vi "poly_fit.vi"(0 "y":dbl[](array[numeric]), 1 "order":i32, 5 "x":dbl[](array[numeric])) -> (4 "P(A)":dbl[](array[numeric]), 6 "P(x)":dbl[](array[numeric]), 15 "error":i32)   [LabVIEW 2020]
uses:
  <vilib>/Analysis/Matrix/Numeric/Conversions/Array To Matrix - RA.vi
  <vilib>/Analysis/Matrix/Numeric/Conversions/Array To Matrix - RA2.vi
  <vilib>/Analysis/Matrix/Numeric/Multiply/Multiply - RM,RM.vi
  <vilib>/Analysis/baseanly.llb/Real Inverse Matrix.vi
  <vilib>/Analysis/Matrix/Numeric/Conversions/Matrix To Array - RM.vi
  <vilib>/Analysis/Matrix/NI_Matrix.lvlib
  <vilib>/Analysis/NI_AALBase.lvlib
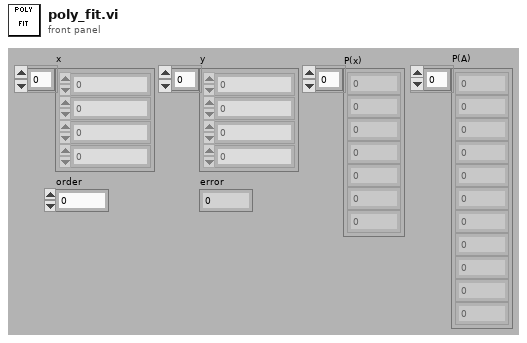
[diagram p1: front panel]
types:
  T1 = typedef "NI_Matrix.lvlib/RealMatrix.ctl" = dbl[][]
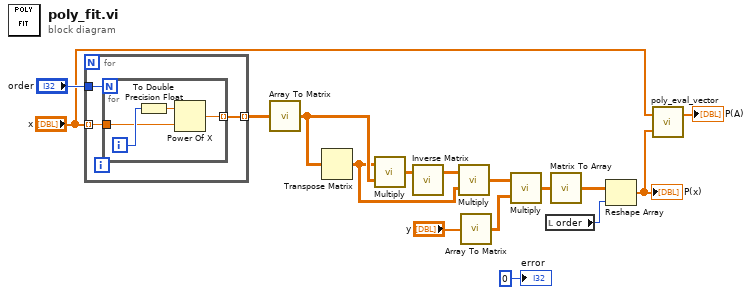
[diagram p0: block diagram]
diagram:
  n1 = for {
    tunnel: "x" -> [w19] mode=indexing
    tunnel: [w18] -> w16 mode=indexing
    tunnel: "order" -> [w17]
    n2 = for {
      N: w17 -> [_]
      tunnel: w19 -> [w21]
      tunnel: [w20] -> w18 mode=indexing
      i -> [w22]
      n3 = To Double Precision Float(number=w22) -> (double precision float=w23:dbl)
      n4 = Power Of X(1:w21, 2:w23) -> (0:w20:dbl)
    }
  }
  n5 = call-poly <vilib>:"Array To Matrix.vi"("Real 2D Array"=w16) -> ("Real Matrix"=w15:T1)
  n6 = Transpose Matrix(1:w15) -> (0:w12:T1)
  n7 = call-poly <vilib>:"Multiply.vi"("Real Matrix B"=w15, "Real Matrix A"=w12) -> ("A * B"=w14:T1)
  n8 = call-poly <vilib>:"Inverse Matrix.vi"("Input Matrix"=w14) -> ("Inverse Matrix"=w13:T1)  [unwired: 1 in, 1 out]
  n9 = call-poly <vilib>:"Multiply.vi"("Real Matrix B"=w12, "Real Matrix A"=w13) -> ("A * B"=w10:T1)
  n10 = call-poly <vilib>:"Array To Matrix.vi"("Real 1D Array"="y") -> ("Real Matrix (Column Vector)"=w9:T1)
  n11 = call-poly <vilib>:"Multiply.vi"("Real Matrix B"=w9, "Real Matrix A"=w10) -> ("A * B"=w8:T1)
  n12 = local read "order"() -> (w5:i32)
  n13 = call-poly <vilib>:"Matrix To Array.vi"("Real Matrix"=w8) -> ("Real 2D Array"=w6:dbl[][])
  n14 = Reshape Array(w6, w5) -> (w4:dbl[])
  "P(x)" <- w4
  n15 = call "poly_eval_vector.vi"("P(x)"=w4, "A"="x") -> ("P(A)"=→"P(A)":dbl[])  [unwired: 1 in]
  "error" <- 0 ("error")
